vi "Create All Message Queues.vi"(8 "error in (no error)":errorcluster, 11 "Initiliaze":T1 {"Database"."Balance" format="%#.2f"; "Database"."Account Number" format="%_1f"}) -> (0 "error out":errorcluster, 3 "QMH":T4)   [LabVIEW 2020, in "Message Queue.lvlib"]
doc: "This VI creates and initializes all the message queues for the application."
uses:
  Message Queue.lvlib
  All Message Queues.ctl
  Message Cluster.ctl
  Controls/Data_Initialize.ctl
  Database/Controls/Account Database.ctl
  Controls/Events_User.ctl
  Enqueue Message (Single).vi
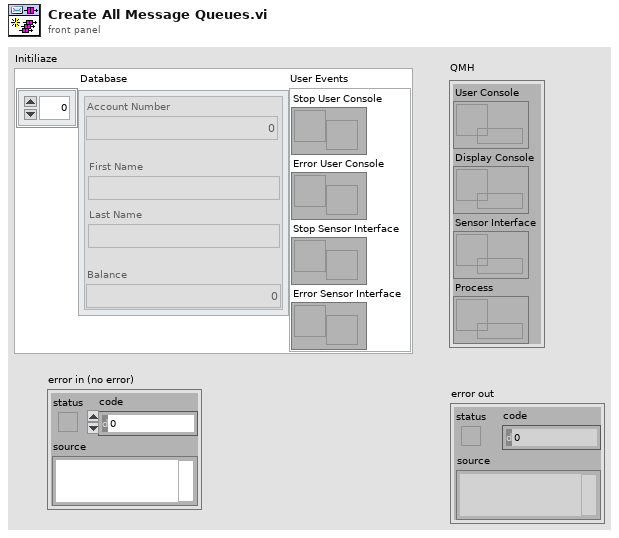
[diagram p1: front panel]
types:
  T1 = typedef "Data_Initialize.ctl" = cluster{"Database":T2[], "User Events":T3}
  T2 = typedef "Account Database.ctl" = cluster{"Account Number":i32, "First Name":string, "Last Name":string, "Balance":dbl}
  T3 = typedef "Events_User.ctl" = cluster{"Stop User Console":refnum<user-event>, "Error User Console":refnum<user-event>, "Stop Sensor Interface ":refnum<user-event>, "Error Sensor Interface":refnum<user-event>}
  T4 = typedef "Message Queue.lvlib/All Message Queues.ctl" = cluster{"User Console":refnum<queue>, "Display Console":refnum<queue>, "Sensor Interface":refnum<queue>, "Process":refnum<queue>}
  T5 = cluster{"[0]":refnum<queue>, "[1]":refnum<queue>, "[2]":refnum<queue>, "[3]":refnum<queue>}
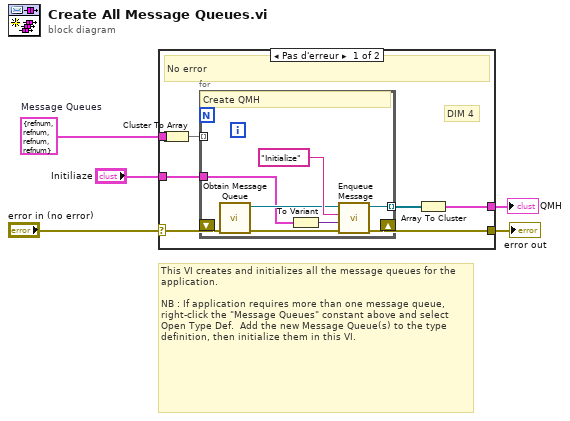
[diagram p0: block diagram]
diagram:
  w1 = T4 {"User Console"=refnum, "Display Console"=refnum, "Sensor Interface"=refnum, "Process"=refnum}  # Message Queues
  # "This VI creates and initializes all the message queues for the application. \n\nNB : If application requires more than one message queue, right-click the \"Message Queues\" constant above and select Open Type Def.  Add the new Message Queue(s) to the type definition, then initialize them in this VI."
  n1 = case shown="Pas d'erreur" "error in (no error)" {
    selector: "error in (no error)" -> [w11 w21]
    tunnel: [w12 w21] -> w5
    tunnel: [w6 _] -> w4
    tunnel: "Initiliaze" -> [w10 _]
    tunnel: w1 -> [w9 _]
    frame No Error {
      # "DIM 4"
      # "No error"
      n2 = Cluster To Array(cluster=w9) -> (array=w8:refnum<queue>[])
      n3 = for {
        tunnel: w10 -> [w15]
        shift-right: [w20] -> w12
        shift-left: w11 -> [w19]
        tunnel: w8 -> [_] mode=indexing
        tunnel: [w13] -> w7 mode=indexing
        # "Create QMH"
        n4 = call "Obtain Message Queue.vi"("error in (no error)"=w19) -> ("error out"=w18:errorcluster, "Message Queue"=w16:refnum<queue>)  [unwired: 9 in]
        n5 = To Variant(anything=w15) -> (Variant=w14:variant)
        n6 = call-poly "Enqueue Message.vi"("error in (no error)"=w18, "Message Data"=w14, "Message"="Initialize", "Message Queue"=w16) -> ("error out"=w20:errorcluster, "dup Message Queue"=w13:refnum<queue>)  [unwired: 6 in]
      }
      n7 = Array To Cluster(array=w7) -> (cluster=w6:T5)
    }
    frame Error {
    }
  }
  "QMH" <- w4
  "error out" <- w5
